vi "Hardcopy.vi"(8 "error in (no error)":errorcluster, 10 "Operation (0: Execute)":u16(ring) items=["Execute", "Abort"], 11 "VISA resource name":refnum<visa-resource-name>) -> (0 "error out":errorcluster, 3 "VISA resource name out":refnum<visa-resource-name>)   [LabVIEW 2018, in "Agilent ENA Series.lvlib"]
doc: "Prints the display image on the LCD display to the printer connected to the E5070B/E5071B/E5071C or abort the print operation.\n\n<b>Note:</b>\nHard Copy Abort is not supported by E5080A."
uses:
  Agilent ENA Series.lvlib
panel:
  # "Note:\nHard Copy Abort is not supported by E5080A."
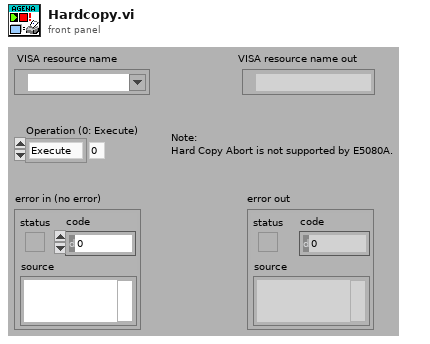
[diagram p1: front panel]
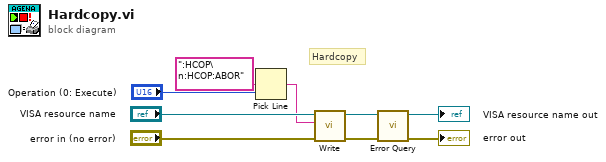
[diagram p0: block diagram]
diagram:
  # "Hardcopy"
  n1 = Pick Line(multi-line string=":HCOP\n:HCOP:ABOR", line index="Operation (0: Execute)") -> (output string=w5:string)  [unwired: 1 in]
  n2 = call "Write.vi"("error in (no error)"="error in (no error)", "String ()"=w5, "VISA resource name"="VISA resource name") -> ("error out"=w1:errorcluster, "VISA resource name out"=w2:refnum<visa-resource-name>)  [unwired: 6 in, 1 out]
  n3 = call "Error Query.vi"("error in (no error)"=w1, "VISA resource name"=w2) -> ("error out"=→"error out":errorcluster, "VISA resource name out"=→"VISA resource name out":refnum<visa-resource-name>)  [unwired: 6 in, 2 out]
